vi "Set LowLimit.vi"(8 "error in":errorcluster, 10 "LowLimit":refnum<class "Value.lvclass">, 11 "DOMAIN in":refnum<class "DOMAIN.lvclass">) -> (0 "error out":errorcluster, 3 "DOMAIN out":refnum<class "DOMAIN.lvclass">)   [LabVIEW 2019, in "Electronic Datasheet.lvlib" / "DOMAIN.lvclass"]
uses:
  DOMAIN.lvclass
  Value/Value.lvclass
  Electronic Datasheet.lvlib
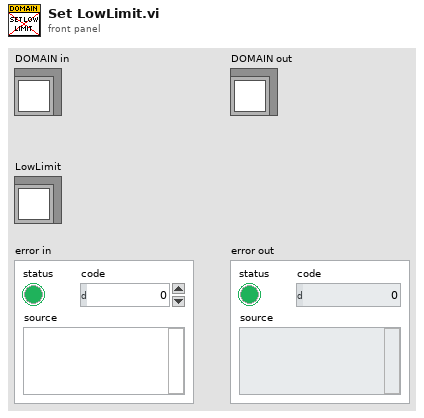
[diagram p1: front panel]
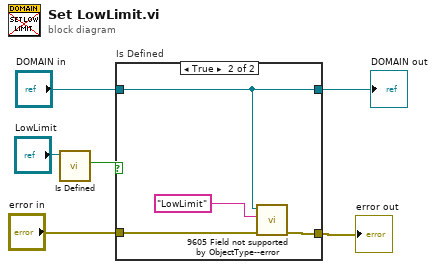
[diagram p0: block diagram]
diagram:
  n1 = call "Is Defined.vi"("Value in"="LowLimit") -> ("Is Defined?"=w1:bool)  [unwired: 9 in, 1 out]
  n2 = case "Is Defined" shown="True" w1 {
    tunnel: "error in" -> [w7 w12]
    tunnel: [w7 w11] -> w5
    tunnel: "DOMAIN in" -> [w8 w9]
    tunnel: [w8 w9] -> w3
    frame False {
    }
    frame True {
      n3 = call "9605 Field not supported by ObjectType--error.vi"("error in"=w12, "Field Name"="LowLimit" ("Field name"), "Object Type Base"=w9) -> ("error out"=w11:errorcluster)  [unwired: 7 in, 1 out]
    }
  }
  "DOMAIN out" <- w3
  "error out" <- w5
